vi "create B scan save path.vi"(9 "B scan index":i32, 10 "Scan Save File Header":string, 11 "Scan Save Path":path) -> (3 "Path":path)   [LabVIEW 2014]
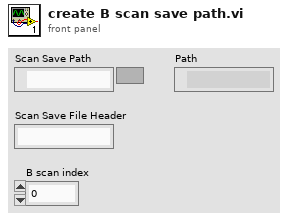
[diagram p1: front panel]
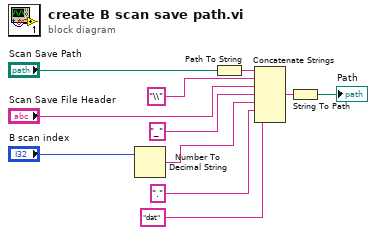
[diagram p0: block diagram]
diagram:
  n1 = Number To Decimal String(number="B scan index") -> (decimal integer string=w9:string)  [unwired: 1 in]
  n2 = Path To String(path="Scan Save Path") -> (string=w2:string)
  n3 = Concatenate Strings(w2, "\\" ("string"), "Scan Save File Header", "_" ("string"), w9, "." ("string"), "dat" ("string")) -> (w6:string)
  n4 = String To Path(string=w6) -> (path=→"Path":path)
